vi "FTW-XML-Element-GetNextSibling.vi"(0 "XML Node":refnum<k20>, 11 "error in":errorcluster) -> (4 "XML Node out":refnum<k20>, 6 "Next Sibling":refnum<k20>, 8 "Found?":bool, 15 "error out":errorcluster)   [LabVIEW 2012]
uses:
  <resource>/objmgr/DOMUserDefRef.rc
panel:
  # "Inputs"
  # "Outputs"
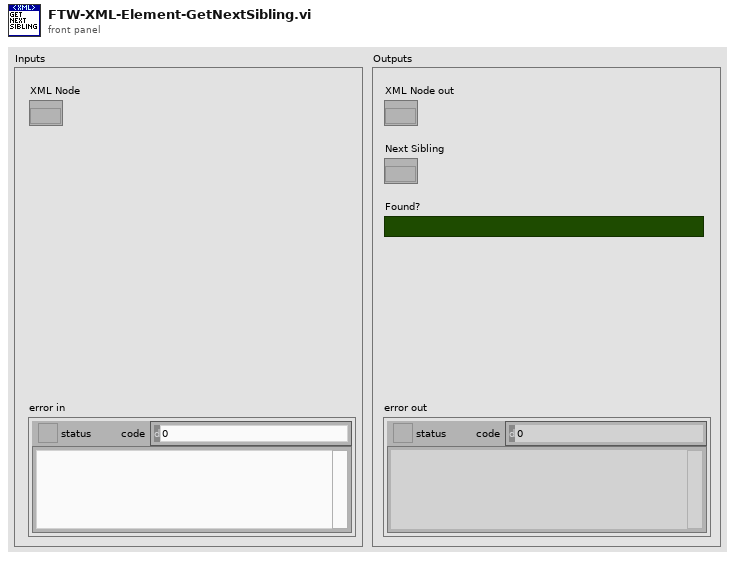
[diagram p1: front panel]
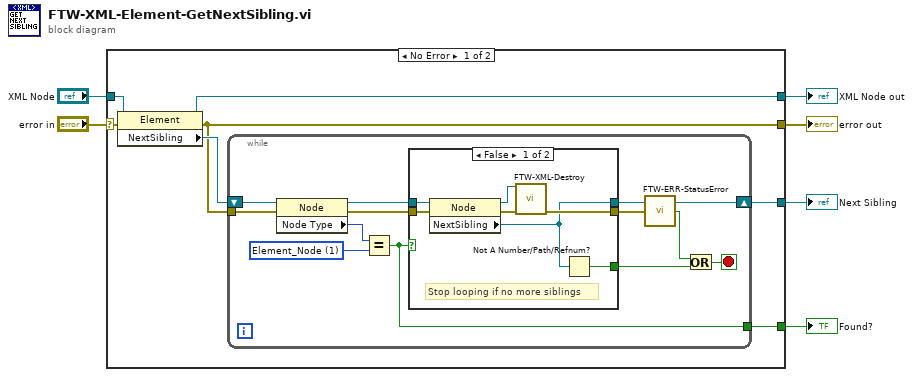
[diagram p0: block diagram]
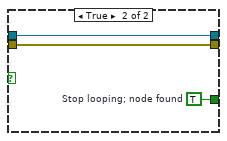
[diagram p2: hidden frame]
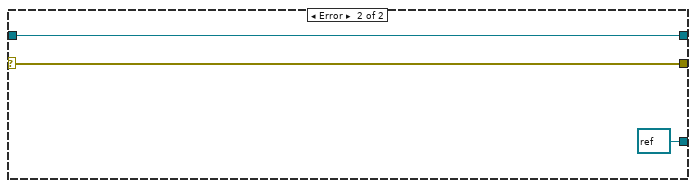
[diagram p3: hidden frame]
diagram:
  n1 = case shown="No Error" "error in" {
    selector: "error in" -> [w11 w38]
    tunnel: [w7 w38] -> w6
    tunnel: "XML Node" -> [w13 w37]
    tunnel: [w12 w37] -> w3
    tunnel: [w9 refnum<k20> refnum ("NextSibling")] -> w2
    tunnel: [w8 _] -> w1
    frame No Error {
      n2 = property class="Element"(reference=w13, error in=w11) -> (reference out=w12:refnum<k20>, error out=w7:errorcluster, "NextSibling"=w10:refnum<k20>)
      n3 = while {
        shift-right: [w20] -> w9
        shift-left: w10 -> [w24]
        tunnel: [w14] -> w8
        tunnel: w7 -> [w25]
        stop <- w16 stop-if-true
        w22 = 1 items=["Element_Node"=1, "Attribute_Node"=2, "Text_Node"=3, "CDATASection_Node"=4, "EntityReference_Node"=5, "Entity_Node"=6, "ProcessingInstruction_Node"=7, "Comment_Node"=8, "Document_Node"=9, "DocumentType_Node"=10, "DocumentFragment_Node"=11, "Notation_Node"=12] ("Node Type")
        n4 = property class="Node"(reference=w24, error in=w25) -> (reference out=w21:refnum<k20>, error out=w19:errorcluster, "Node Type"=w23:i32)
        n5 = Equal?(x=w23, y=w22) -> (x = y?=w14:bool)
        n6 = case shown="False" w14 {
          tunnel: w21 -> [w32 w35]
          tunnel: [w27 w35] -> w20
          tunnel: w19 -> [w31 w34]
          tunnel: [w28 w34] -> w18
          tunnel: [w26 w33] -> w15
          frame False {
            # "Stop looping if no more siblings"
            n7 = property class="Node"(reference=w32, error in=w31) -> (reference out=w29:refnum<k20>, error out=w30:errorcluster, "NextSibling"=w27:refnum<k20>)
            n8 = call "FTW-XML-Destroy.vi"("XML Node"=w29, "error in"=w30) -> ("error out"=w28:errorcluster)  [unwired: 13 in]
            n9 = Not A Number/Path/Refnum?(number/path/refnum=w27) -> (NaN/Path/Refnum?=w26:bool)
          }
          frame True {
            w33 = TRUE  # Stop looping; node found
          }
        }
        n10 = call "FTW-ERR-StatusError.vi"("error to check"=w18) -> ("Error?"=w17:bool)
        n11 = Or(x=w17, y=w15) -> (x .or. y?=w16:bool)
      }
    }
    frame Error {
    }
  }
  "error out" <- w6
  "XML Node out" <- w3
  "Found?" <- w1
  "Next Sibling" <- w2
